vi "Handle Error Event.vi"(6 "error source":T1, 8 "error in":errorcluster, 9 "data":variant, 10 "event":variant, 11 "module reference in":T2) -> (0 "error out":errorcluster, 3 "module reference out":T2)   [LabVIEW 2017, in "Controller.lvlib"]
uses:
  Controller.lvlib
  Private TypeDefs/Module Reference.ctl
  Global TypeDefs/Registered Modules.ctl
  Private TypeDefs/Module Queues.ctl
  Private TypeDefs/Message Queue Element.ctl
  Private TypeDefs/Messages.ctl
  Private TypeDefs/Module Notifiers.ctl
  Private TypeDefs/Dummy Notifier.ctl
  Private TypeDefs/Event and Data.ctl
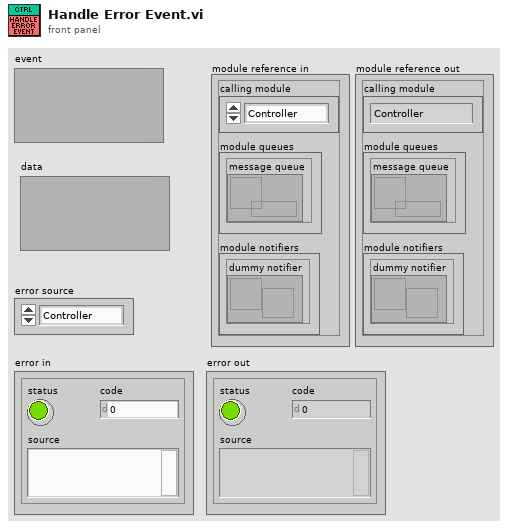
[diagram p1: front panel]
types:
  T1 = typedef "Registered Modules.ctl" = enum16{"Controller", "DAQ", "Error Handler", "Game", "myPAM", "WinHost", "Logger"}
  T2 = typedef "Controller.lvlib/Module Reference.ctl" = cluster{"calling module":T1, "module queues":T3, "module notifiers":T4}
  T3 = typedef "Controller.lvlib/Module Queues.ctl" = cluster{"message queue":refnum<queue>}
  T4 = typedef "Controller.lvlib/Module Notifiers.ctl" = cluster{"dummy notifier":refnum<notifier>}
  T5 = typedef "Controller.lvlib/Messages.ctl" = enum16{"shutdown", "handle event", "start system"}
  T6 = typedef "Controller.lvlib/Event and Data.ctl" = cluster{"event":variant, "data":variant}
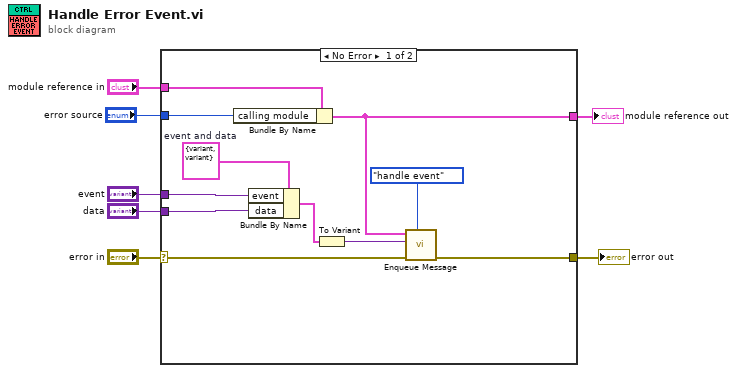
[diagram p0: block diagram]
diagram:
  n1 = case shown="No Error" "error in" {
    selector: "error in" -> [w18 w20]
    tunnel: [w11 w20] -> w2
    tunnel: "module reference in" -> [w10 w19]
    tunnel: [w8 w19] -> w5
    tunnel: "event" -> [w15 _]
    tunnel: "data" -> [w14 _]
    tunnel: "error source" -> [w9 _]
    frame No Error {
      w16 = T6 {"event"=variant, "data"=variant}  # event and data
      n2 = Bundle By Name(cluster=w10, "calling module"=w9) -> (w8:T2)
      n3 = Bundle By Name(cluster=w16, "event"=w15, "data"=w14) -> (w13:T6)
      n4 = To Variant(anything=w13) -> (Variant=w12:variant)
      n5 = call "Enqueue Message.vi"("message"=Messages."handle event", "error in"=w18, "data"=w12, "module reference in"=w8) -> ("error out"=w11:errorcluster)  [unwired: 6 in, 1 out]
    }
    frame Error {
    }
  }
  "module reference out" <- w5
  "error out" <- w2
